vi "Destroy.vi"(8 "error in (no error)":errorcluster, 11 "SignalGeneratorService in":refnum<class "iService.lvclass">) -> (0 "error out":errorcluster, 3 "SignalGeneratorService out":refnum<class "iService.lvclass">)   [LabVIEW 2019, in "gRPC-servicer.lvlib" / "iService.lvclass"]
uses:
  iService.lvclass
  iService.lvclass/iService.ctl
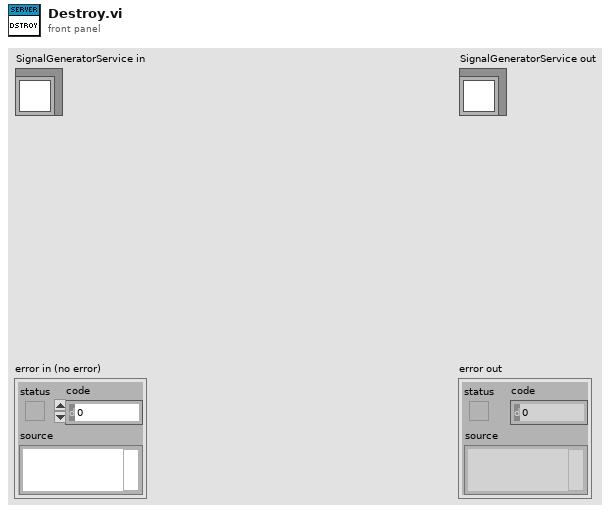
[diagram p1: front panel]
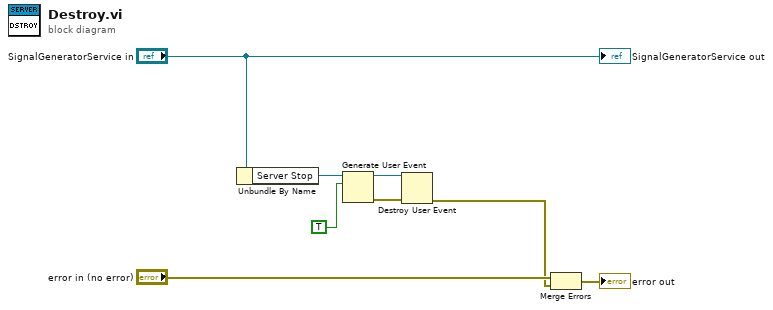
[diagram p0: block diagram]
diagram:
  n1 = Unbundle By Name("SignalGeneratorService in") -> ("Server Stop"=w6:refnum<user-event>)
  n2 = Generate User Event(user event=w6, event data cluster=TRUE) -> (user event out=w4:refnum<user-event>, error out=w5:errorcluster)  [unwired: 2 in]
  n3 = Destroy User Event(user event=w4, error in=w5) -> (error out=w1:errorcluster)
  n4 = Merge Errors("error in (no error)", w1) -> (→"error out":errorcluster)
  "SignalGeneratorService out" <- "SignalGeneratorService in"
